vi "Search Account.vi"(8 "error in":errorcluster, 10 "Account Number":i32 format="%_1f", 11 "Database IN":T1[](array[typedef]) {"Balance" format="%#.2f"; "Account Number" format="%_1f"}) -> (0 "error out":errorcluster, 2 "Index Account":i32, 3 "Configuration Database":T1 {"Balance" format="%#.2f"; "Account Number" format="%_1f"})   [LabVIEW 2020]
doc: "Search account VI provide account data and index based on account number"
uses:
  Controls/Account Database.ctl
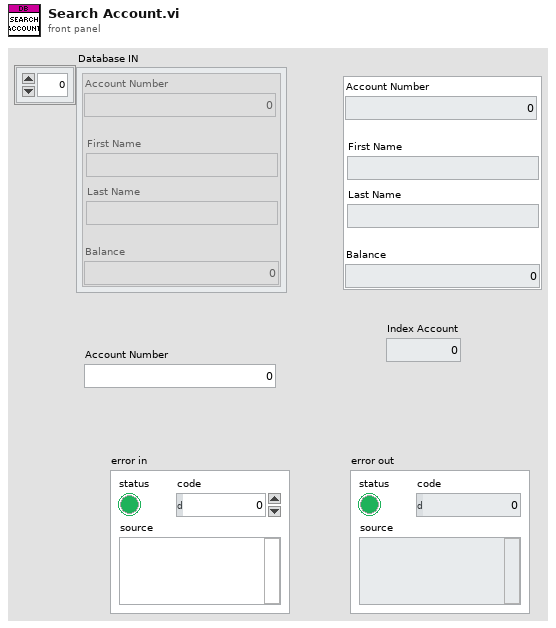
[diagram p1: front panel]
types:
  T1 = typedef "Account Database.ctl" = cluster{"Account Number":i32, "First Name":string, "Last Name":string, "Balance":dbl}
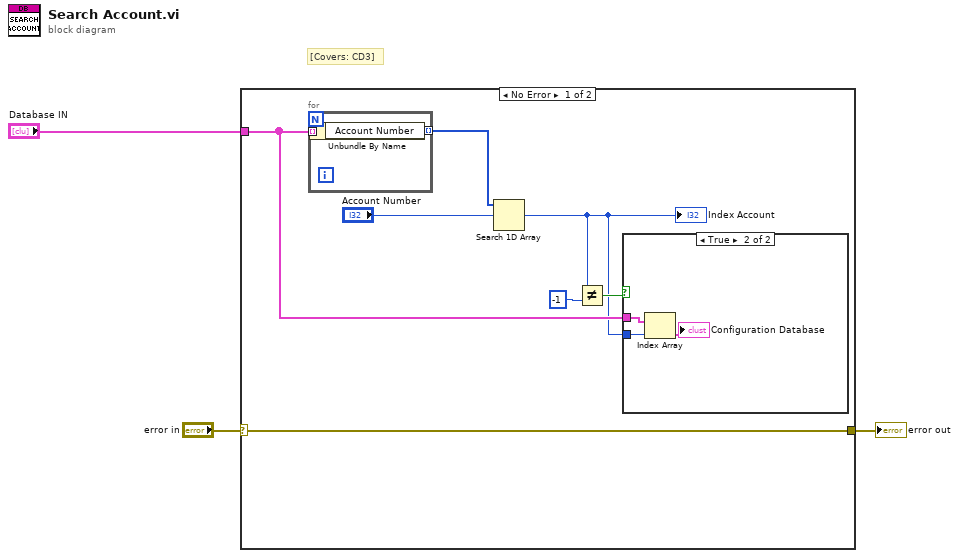
[diagram p0: block diagram]
diagram:
  # "[Covers: CD3]"
  n1 = case shown="No Error" "error in" {
    selector: "error in" -> [w10 w16]
    tunnel: [w10 w16] -> w2
    tunnel: "Database IN" -> [w5 _]
    frame No Error {
      n2 = for {
        tunnel: w5 -> [w15] mode=indexing
        tunnel: [w14] -> w9 mode=indexing
        n3 = Unbundle By Name(w15) -> ("Account Number"=w14:i32)
      }
      n4 = Search 1D Array(1D array=w9, element="Account Number") -> (index of element=w4:i32)  [unwired: 1 in]
      "Index Account" <- w4
      n5 = Not Equal?(x=w4, y=-1) -> (x != y?=w6:bool)
      n6 = case shown="True" w6 {
        tunnel: w5 -> [_ w13]
        tunnel: w4 -> [_ w11]
        frame False {
        }
        frame True {
          n7 = Index Array(array=w13, index=w11) -> (element=→"Configuration Database":T1)
        }
      }
    }
    frame Error {
    }
  }
  "error out" <- w2
